vi "Send OOB TX.vi"(8 "error in (no error)":errorcluster, 11 "CIFCorePlugin in":refnum<class "CIFCorePlugin.lvclass">) -> (0 "error out":errorcluster, 3 "CIFCorePlugin out":refnum<class "CIFCorePlugin.lvclass">)   [LabVIEW 2021, in "CIFCorePlugin.lvclass"]
uses:
  CIFCorePlugin.lvclass
  CIFCorePlugin.lvclass/CIFCorePlugin.ctl
  CIFCoreCommon/Typedef/Plugin Status.ctl
  CIFCoreCommon/Typedef/Plugin State.ctl
  CIFCoreCommon/Typedef/Timing Statistics.ctl
  CIFCoreCommon/Typedef/Timing Stats Base.ctl
  CIFCoreCommon/Typedef/FIFO Statistics.ctl
  CIFCoreCommon/Typedef/Simple Error.ctl
  CIFCoreCommon/Typedef/Monitor Doubles.ctl
  CIFCoreCommon/Typedef/Monitor U64.ctl
  CIFCoreCommon/Typedef/Monitor I64.ctl
  CIFCoreCommon/Typedef/Plugin Overrides.ctl
  CIFCoreCommon/Typedef/Timing Overrides.ctl
  CIFUtilities/CIFOutOfBand/CIFOutOfBand.lvclass/CIFOutOfBand.ctl
  CIFUtilities/CIFOutOfBand/Write OOB DVR.vi
  CIFUtilities/CIFOutOfBand/Utilities/Command to Bitwise Command.vi
  CIFUtilities/CIFOutOfBand/Accessors/Read Local OOB Data.vi
  CIFUtilities/CIFOutOfBand/Accessors/Write Local OOB Data.vi
  CIFCoreOOB/OOB_Tx/CIFCoreOOB_Tx.lvclass
  D:/dev/CIF-LVCore/src/CIFUtilities/CIFOutOfBand/CIFOutOfBand.lvclass
  CIFCoreCommon/CIFCoreCommon.lvlib
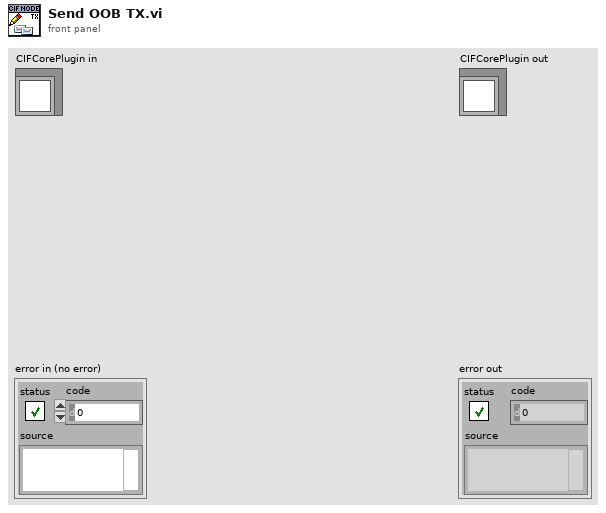
[diagram p1: front panel]
types:
  T1 = typedef "CIFCoreCommon.lvlib/Plugin Overrides.ctl" = cluster{"Timing Overrides":T2}
  T2 = typedef "CIFCoreCommon.lvlib/Timing Overrides.ctl" = cluster{"Override Timing":bool, "Period (s)":dbl}
  T3 = typedef "CIFCoreCommon.lvlib/Plugin Status.ctl" = cluster{"State":T4, "Timing Statistics (us)":T5, "FIFO Statistics (us)":T7, "error":T8, "Monitor Doubles":T9, "Monitor U64":T10, "Monitor I64":T11}
  T4 = typedef "CIFCoreCommon.lvlib/Plugin State.ctl" = enum32{"Null", "Creating", "Listening", "Running", "CleaningUp", "Destroying"}
  T5 = typedef "CIFCoreCommon.lvlib/Timing Statistics.ctl" = cluster{"Period":T6, "Wake Error":T6, "Execute":T6, "Housekeep":T6, "Idle":T6}
  T6 = typedef "CIFCoreCommon.lvlib/Timing Stats Base.ctl" = cluster{"Max":i32, "Min":i32}
  T7 = typedef "CIFCoreCommon.lvlib/FIFO Statistics.ctl" = cluster{"From T0":T6, "From Previous Plugin":T6, "Output Error":T6}
  T8 = typedef "CIFCoreCommon.lvlib/Simple Error.ctl" = cluster{"status":bool, "code":i32}
  T9 = typedef "CIFCoreCommon.lvlib/Monitor Doubles.ctl" = cluster{"1":dbl, "2":dbl, "3":dbl, "4":dbl}
  T10 = typedef "CIFCoreCommon.lvlib/Monitor U64.ctl" = cluster{"1":u64, "2":u64, "3":u64, "4":u64}
  T11 = typedef "CIFCoreCommon.lvlib/Monitor I64.ctl" = cluster{"1":i64, "2":i64, "3":i64, "4":i64}
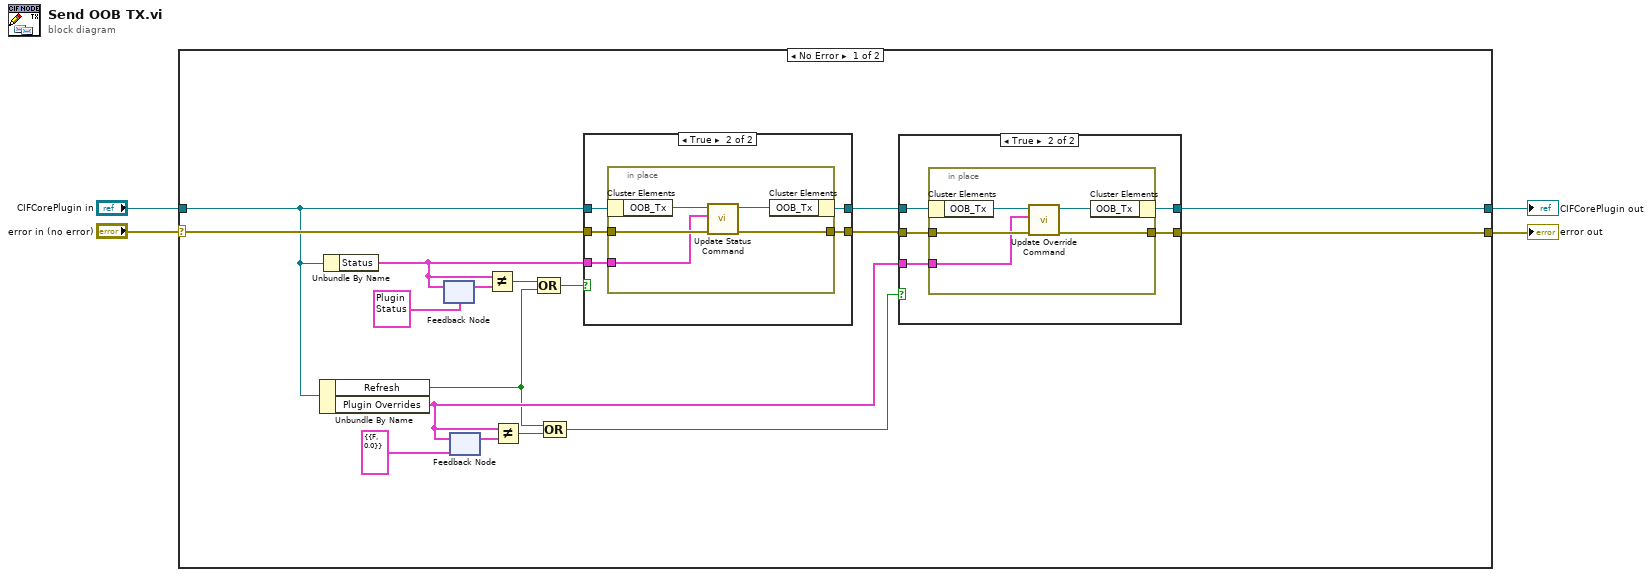
[diagram p0: block diagram]
diagram:
  n1 = case shown="No Error" "error in (no error)" {
    selector: "error in (no error)" -> [w21 w47]
    tunnel: [w13 w47] -> w3
    tunnel: [w5 w46] -> w1
    tunnel: "CIFCorePlugin in" -> [w12 w46]
    frame No Error {
      n2 = Unbundle By Name(w12) -> ("Refresh"=w6:bool, "Plugin Overrides"=w7:T1)
      n3 = Unbundle By Name(w12) -> ("Status"=w17:T3)
      n4 = feedback-in #1(w17) -> ()
      n5 = feedback #1(T3 {"State"=enum."Null", "Timing Statistics (us)"={"Period"={"Max"=0, "Min"=0}, "Wake Error"={"Max"=0, "Min"=0}, "Execute"={"Max"=0, "Min"=0}, "Housekeep"={"Max"=0, "Min"=0}, "Idle"={"Max"=0, "Min"=0}}, "FIFO Statistics (us)"={"From T0"={"Max"=0, "Min"=0}, "From Previous Plugin"={"Max"=0, "Min"=0}, "Output Error"={"Max"=0, "Min"=0}}, "error"={"status"=FALSE, "code"=0}, "Monitor Doubles"={"1"=0.0, "2"=0.0, "3"=0.0, "4"=0.0}, "Monitor U64"={"1"=0, "2"=0, "3"=0, "4"=0}, "Monitor I64"={"1"=0, "2"=0, "3"=0, "4"=0}} ("Status")) -> (w19:T3)
      n6 = feedback #2(T1 {"Timing Overrides"={"Override Timing"=FALSE, "Period (s)"=0.0}} ("Plugin Overrides")) -> (w10:T1)
      n7 = feedback-in #2(w7) -> ()
      n8 = Not Equal?(x=w17, y=w19) -> (x != y?=w18:bool)
      n9 = Not Equal?(x=w7, y=w10) -> (x != y?=w11:bool)
      n10 = Compound Arithmetic op=OR(w18, w6) -> (w16:bool)
      n11 = Compound Arithmetic op=OR(w6, w11) -> (w8:bool)
      n12 = case shown="True" w16 {
        tunnel: w21 -> [w34 w40]
        tunnel: w12 -> [w35 w39]
        tunnel: w17 -> [_ w38]
        tunnel: [w35 w37] -> w15
        tunnel: [w34 w36] -> w14
        frame False {
        }
        frame True {
          n13 = in-place {
            in-place-border: w40 -> [w43]
            in-place-border: [w42] -> w36
            in-place-border: w38 -> [w41]
            n14 = in-place-cluster #3(w39) -> ("OOB_Tx"=w45:refnum<class "CIFCoreOOB_Tx.lvclass">)
            n15 = call "Update Status Command.vi"("error in"=w43, "Status"=w41, "CoreOOB_Tx in"=w45) -> ("error out"=w42:errorcluster, "CoreOOB_Tx out"=w44:refnum<class "CIFCoreOOB_Tx.lvclass">)  [unwired: 7 in]
            n16 = in-place-cluster #3("OOB_Tx"=w44) -> (w37:refnum<class "CIFCorePlugin.lvclass">)
          }
        }
      }
      n17 = case shown="True" w8 {
        tunnel: w14 -> [w22 w28]
        tunnel: w15 -> [w23 w27]
        tunnel: w7 -> [_ w26]
        tunnel: [w23 w25] -> w5
        tunnel: [w22 w24] -> w13
        frame False {
        }
        frame True {
          n18 = in-place {
            in-place-border: w28 -> [w31]
            in-place-border: [w30] -> w24
            in-place-border: w26 -> [w29]
            n19 = in-place-cluster #4(w27) -> ("OOB_Tx"=w33:refnum<class "CIFCoreOOB_Tx.lvclass">)
            n20 = call "Update Override Command.vi"("error in"=w31, "Plugin Overrides"=w29, "CoreOOB_Tx in"=w33) -> ("error out"=w30:errorcluster, "CoreOOB_Tx out"=w32:refnum<class "CIFCoreOOB_Tx.lvclass">)  [unwired: 7 in]
            n21 = in-place-cluster #4("OOB_Tx"=w32) -> (w25:refnum<class "CIFCorePlugin.lvclass">)
          }
        }
      }
    }
    frame Error {
    }
  }
  "error out" <- w3
  "CIFCorePlugin out" <- w1
